vi "Dequeue Event Message by Sender.vi"(8 "error in (no error)":errorcluster, 9 "Timeout (-1)":i32=-1, 10 "Sender":string, 11 "Event Registration Refnum":refnum<event-registration>) -> (0 "error out":errorcluster, 1 "Message Data":variant, 2 "Message":string, 3 "Event Registration Refnum Out":refnum<event-registration>, 4 "Timed Out?":bool)   [LabVIEW 2020, in "Framework Test Support.lvlib" / "Event Helpers.lvlib"]
uses:
  Event Helpers.lvlib
  Framework/Process/Protected/Broadcasting/Broadcast Message Cluster.ctl
  Framework Test Support.lvlib
  Framework/Process/Process.lvclass
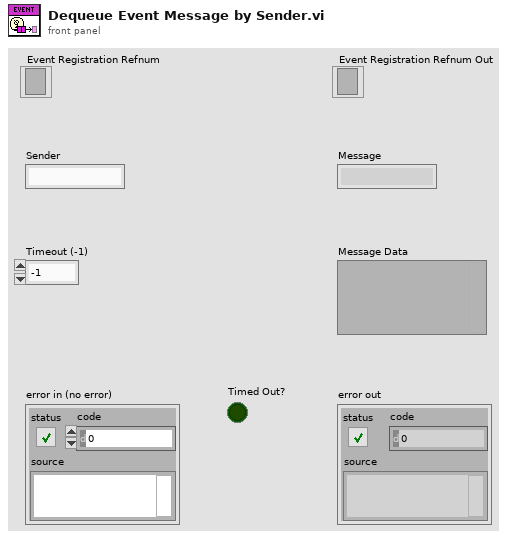
[diagram p1: front panel]
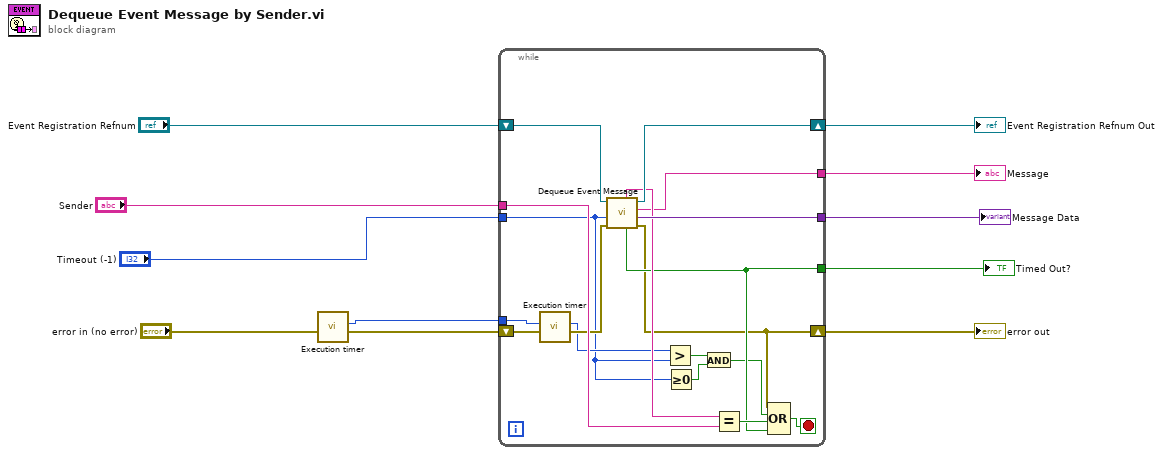
[diagram p0: block diagram]
diagram:
  n1 = call "Execution timer.vi"("error in (no error)"="error in (no error)") -> ("error out"=w2:errorcluster, "Current or Duration [ms]"=w1:u32)  [unwired: 9 in]
  n2 = while {
    tunnel: [w22] -> w7
    tunnel: [w26] -> w6
    tunnel: [w20] -> w5
    tunnel: "Timeout (-1)" -> [w12]
    shift-right: [w28] -> w10
    shift-left: "Event Registration Refnum" -> [w29]
    shift-right: [w15] -> w8
    shift-left: w2 -> [w27]
    tunnel: "Sender" -> [w25]
    tunnel: w1 -> [w18]
    stop <- w21 stop-if-true
    n3 = call "Execution timer.vi"("error in (no error)"=w27, "millisecond timer value"=w18) -> ("error out"=w19:errorcluster, "Current or Duration [ms]"=w13:u32)  [unwired: 8 in]
    n4 = call "Dequeue Event Message.vi"("error in (no error)"=w19, "Timeout (-1)"=w12, "Event Registration Refnum"=w29) -> ("error out"=w15:errorcluster, "Message Data"=w26:variant, "Message"=w22:string, "Event Registration Refnum Out"=w28:refnum<event-registration>, "Timed Out?"=w20:bool, "Sender"=w23:string)  [unwired: 3 in]
    n5 = Greater?(x=w13, y=w12) -> (0:w17:bool)
    n6 = Greater Or Equal To 0?(x=w12) -> (x >= 0?=w16:bool)
    n7 = And(x=w17, y=w16) -> (x .and. y?=w14:bool)
    n8 = Equal?(x=w23, y=w25) -> (x = y?=w24:bool)
    n9 = Compound Arithmetic op=OR(w15, w14, w24, w20) -> (w21:bool)
  }
  "Event Registration Refnum Out" <- w10
  "Message Data" <- w6
  "Message" <- w7
  "error out" <- w8
  "Timed Out?" <- w5
